vi "PID Integral Action (DBL).vi"(4 "output range":cluster{"output high":dbl, "output low":dbl}={"output high"=100.0, "output low"=-100.0} {"output low" format="%.2f"; "output high" format="%.2f"}, 5 "error":dbl format="%.2f", 6 "dt (min)":dbl format="%.3f", 7 "proportional action":dbl format="%.2f", 8 "initialize (F)":bool, 9 "derivative action":dbl format="%.2f", 10 "PID gains":T1={"proportional gain (Kc)"=1.0, "integral time (Ti, min)"=0.01, "derivative time (Td, min)"=0.0} {"derivative time (Td, min)" format="%.3f"; "integral time (Ti, min)" format="%.3f"; "proportional gain (Kc)" format="%.3f"}, 11 "Ki":dbl format="%.2f") -> (3 "output":dbl format="%.2f")   [LabVIEW 2020, in "NI_PID_pid.lvlib"]
uses:
  NI_PID_pid.lvlib
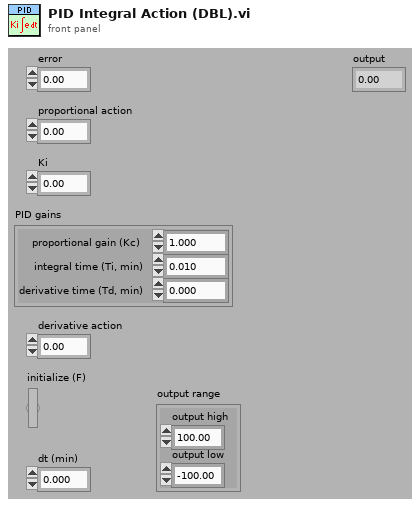
[diagram p1: front panel]
types:
  T1 = cluster{"proportional gain (Kc)":dbl, "integral time (Ti, min)":dbl, "derivative time (Td, min)":dbl}
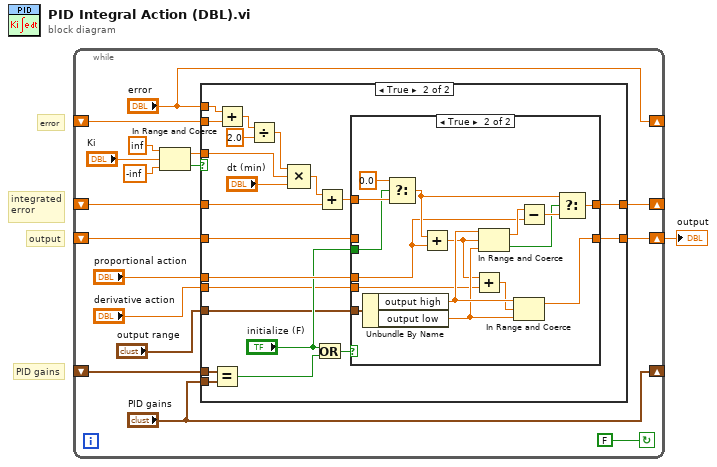
[diagram p0: block diagram]
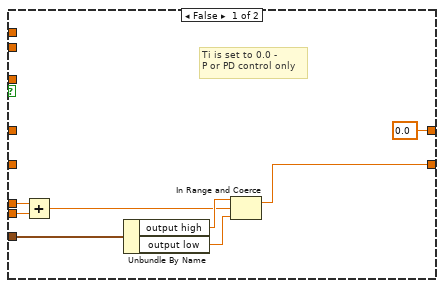
[diagram p2: hidden frame]
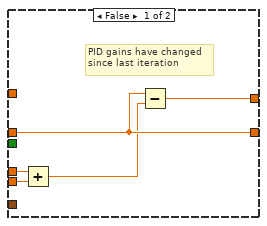
[diagram p3: hidden frame]
diagram:
  # "PID gains"
  # "output"
  # "integrated\nerror"
  # "error"
  n1 = while {
    shift-left: _ -> [w7]
    shift-right: [w6] -> w1
    shift-left: _ -> [w17]
    shift-right: ["error"] -> _
    shift-left: _ -> [w16]
    shift-right: [w15] -> _
    shift-left: _ -> [w10]
    shift-right: ["PID gains"] -> _
    stop <- FALSE continue-if-true
    n2 = In Range and Coerce(upper limit=inf, x="Ki", lower limit=-inf) -> (coerced(x)=w5:dbl, In Range?=w11:bool)
    n3 = case shown="True" w11 {
      tunnel: "error" -> [_ w46]
      tunnel: w17 -> [_ w47]
      tunnel: w16 -> [_ w41]
      tunnel: [0.0 ("t") w31] -> w15
      tunnel: w5 -> [_ w29]
      tunnel: "proportional action" -> [w21 w39]
      tunnel: w10 -> [_ w37]
      tunnel: "PID gains" -> [_ w36]
      tunnel: [w26 w30] -> w6
      tunnel: "output range" -> [w25 w32]
      tunnel: w7 -> [_ w34]
      tunnel: "derivative action" -> [w20 w27]
      frame False {
        # "Ti is set to 0.0 -\nP or PD control only"
        n4 = Add(x=w21, y=w20) -> (x+y=w19:dbl)
        n5 = Unbundle By Name(w25) -> ("output high"=w24:dbl, "output low"=w23:dbl)
        n6 = In Range and Coerce(upper limit=w24, x=w19, lower limit=w23) -> (coerced(x)=w26:dbl)  [unwired: 1 out]
      }
      frame True {
        n7 = Equal?(x=w37, y=w36) -> (x = y?=w38:bool)
        n8 = Add(x=w46, y=w47) -> (x+y=w44:dbl)
        n9 = Divide(x=w44, y=2.0) -> (x/y=w43:dbl)
        n10 = Compound Arithmetic op=MULTIPLY(w43, w29, "dt (min)") -> (w42:dbl)
        n11 = Or(x="initialize (F)", y=w38) -> (x .or. y?=w35:bool)
        n12 = Add(x=w42, y=w41) -> (x+y=w40:dbl)
        n13 = case shown="True" w35 {
          tunnel: w40 -> [_ w59]
          tunnel: w39 -> [w50 w55]
          tunnel: w34 -> [w52 _]
          tunnel: "initialize (F)" -> [_ w58]
          tunnel: w32 -> [_ w53]
          tunnel: [w51 w57] -> w31
          tunnel: [w52 w56] -> w30
          tunnel: w27 -> [w49 w54]
          frame False {
            # "PID gains have changed\nsince last iteration"
            n14 = Add(x=w50, y=w49) -> (x+y=w48:dbl)
            n15 = Subtract(x=w52, y=w48) -> (x-y=w51:dbl)
          }
          frame True {
            n16 = Unbundle By Name(w53) -> ("output high"=w66:dbl, "output low"=w65:dbl)
            n17 = Select(t=0.0, s=w58, f=w59) -> (s? t:f=w62:dbl)
            n18 = Add(x=w62, y=w55) -> (x+y=w61:dbl)
            n19 = Add(x=w61, y=w54) -> (x+y=w60:dbl)
            n20 = In Range and Coerce(upper limit=w66, x=w61, lower limit=w65) -> (coerced(x)=w64:dbl, In Range?=w63:bool)
            n21 = In Range and Coerce(upper limit=w66, x=w60, lower limit=w65) -> (coerced(x)=w56:dbl)  [unwired: 1 out]
            n22 = Subtract(x=w64, y=w55) -> (x-y=w67:dbl)
            n23 = Select(t=w62, s=w63, f=w67) -> (s? t:f=w57:dbl)
          }
        }
      }
    }
  }
  "output" <- w1
